vi "Creat ChildNode.vi"(8 "error in":errorcluster caption="错误输入（无错误）", 11 "ParentDataNode in":refnum<class "PanelDataNode.lvclass"> caption="DNL_LabVIEW Object in") -> (0 "error out":errorcluster caption="错误输出", 2 "ChildDataNode[]":refnum<data-value>[](array[refnum]), 3 "ParentDataNode out":refnum<class "PanelDataNode.lvclass"> caption="DNL_LabVIEW Object out")   [LabVIEW 2013, in "PanelDataNode.lvclass"]
uses:
  PanelDataNode.lvclass
  PanelObject/PanelObject.lvclass
  PanelLinkNode/PanelLinkNode.lvclass/PanelLinkNode.ctl
  PanelLinkNode/PanelLinkNode.lvclass
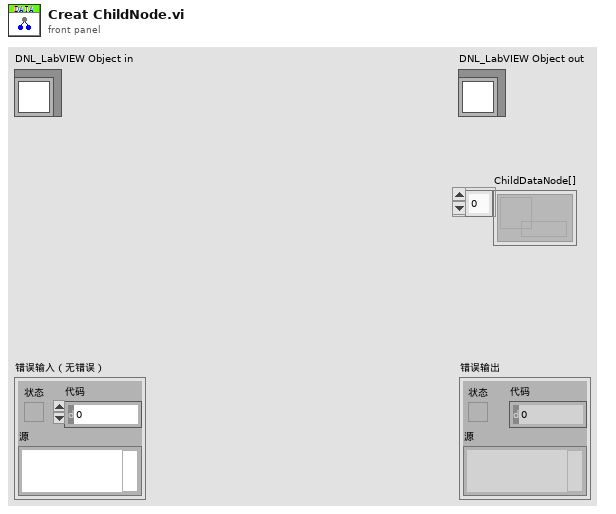
[diagram p1: front panel]
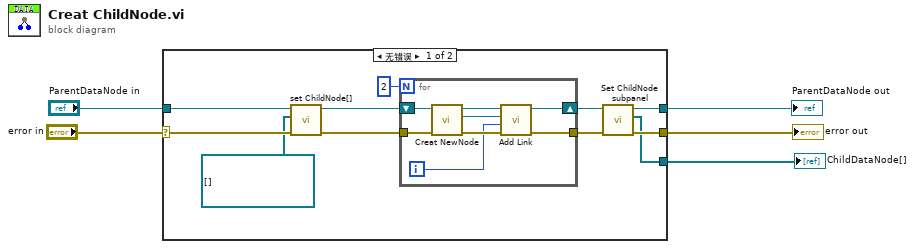
[diagram p0: block diagram]
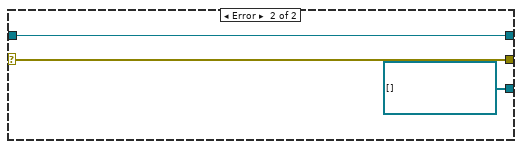
[diagram p2: hidden frame]
diagram:
  n1 = case shown="无错误" "error in" {
    selector: "error in" -> [w14 w27]
    tunnel: [w7 w27] -> w4
    tunnel: [w8 w26] -> w2
    tunnel: "ParentDataNode in" -> [w16 w26]
    tunnel: [w6 refnum<data-value>[] [] ("ChildDataNode[]")] -> w1
    frame No Error {
      n2 = call "set ChildNode[].vi"("error in (no error)"=w14, "ChildNode*[]"=refnum<data-value>[] [], "PanelLinkNode输入"=w16) -> ("error out"=w13:errorcluster, "PanelLinkNode输出"=w15:refnum<class "PanelDataNode.lvclass">)  [unwired: 7 in]
      n3 = for {
        N: 2 -> [_]
        tunnel: [w21] -> w9
        tunnel: w13 -> [w18]
        shift-right: [w20] -> w10
        shift-left: w15 -> [w19]
        i -> [w17]
        n4 = call-dynamic "Creat NewNode.vi"("error in (no error)"=w18, "PanelDataNode 输入"=w19) -> ("error out"=w22:errorcluster, "NewNode*"=w24:refnum<data-value>, "PanelDataNode 输出"=w23:refnum<class "PanelDataNode.lvclass">)  [unwired: 7 in]
        n5 = call-dynamic "Add Link.vi"("ParentLinkNode in"=w23, "ChildNode* in"=w24, "L\\R Child"=w17, "error in (no error)"=w22) -> ("ParentLinkNode out"=w20:refnum<class "PanelDataNode.lvclass">, "error out"=w21:errorcluster)  [unwired: 5 in]
      }
      n6 = call-dynamic "Set ChildNode subpanel.vi"("error in (no error)"=w9, "ParentDataNode in"=w10) -> ("error out"=w7:errorcluster, "ChildDataNode[]"=w6:refnum<data-value>[], "ParentDataNode out"=w8:refnum<class "PanelDataNode.lvclass">)  [unwired: 7 in]
    }
    frame Error {
    }
  }
  "error out" <- w4
  "ParentDataNode out" <- w2
  "ChildDataNode[]" <- w1
